vi "Base Error Code.vi"() -> (3 "base error code":i32)   [LabVIEW 2020, in "RDMA.lvlib" / "RDMA Transceiver.lvclass"]
uses:
  RDMA Transceiver.lvclass
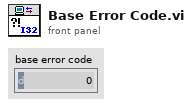
[diagram p1: front panel]
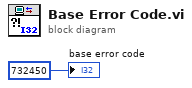
[diagram p0: block diagram]
diagram:
  "base error code" <- 732450 ("base error code")
